vi "generate-folder-name.vi"(7 "vi path base":path, 8 "error in":errorcluster, 9 "report file destination base":path, 11 "vi path":path) -> (0 "error out":errorcluster, 1 "html destination":path, 3 "vi path out":path)   [LabVIEW 2014]
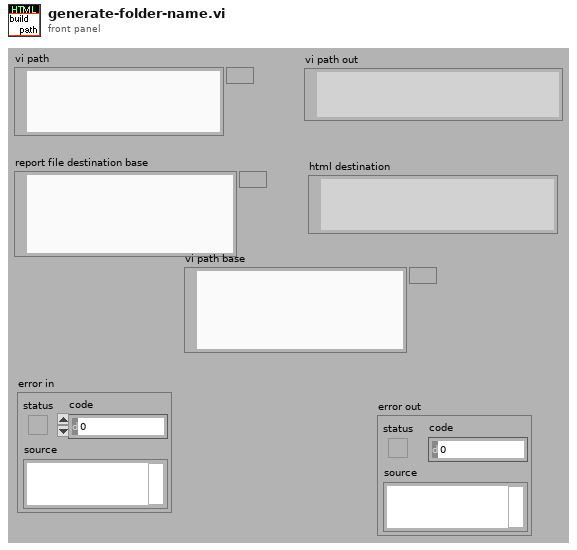
[diagram p1: front panel]
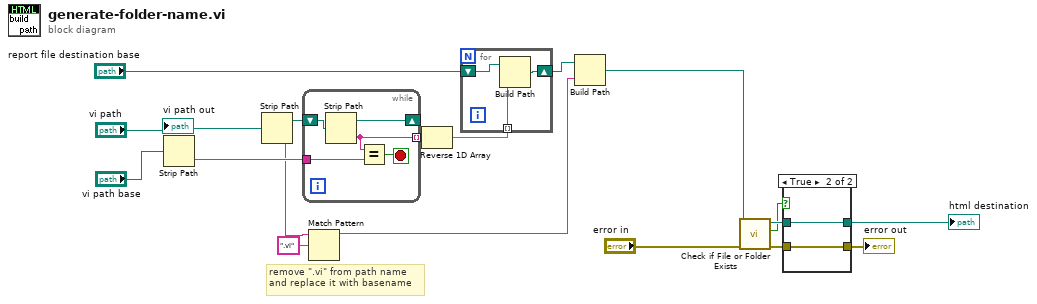
[diagram p0: block diagram]
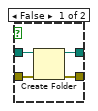
[diagram p2: hidden frame]
diagram:
  # "remove \".vi\" from path name\nand replace it with basename"
  n1 = Strip Path(path="vi path base") -> (name=w12:string)  [unwired: 1 out]
  n2 = Strip Path(path="vi path") -> (stripped path=w9:path, name=w5:string)
  n3 = while {
    shift-right: [w22] -> _
    shift-left: w9 -> [w23]
    tunnel: w12 -> [w21]
    tunnel: [w19] -> w3 mode=indexing
    stop <- w20 stop-if-true
    n4 = Strip Path(path=w23) -> (stripped path=w22:path, name=w19:string)
    n5 = Equal?(x=w19, y=w21) -> (x = y?=w20:bool)
  }
  n6 = Match Pattern(string=w5, regular expression=".vi") -> (before substring=w7:string)  [unwired: 4 out]
  n7 = Reverse 1D Array(array=w3) -> (reversed array=w1:string[])
  n8 = for {
    shift-right: [w25] -> w2
    shift-left: "report file destination base" -> [w26]
    tunnel: w1 -> [w24] mode=indexing
    n9 = Build Path(base path=w26, name or relative path=w24) -> (appended path=w25:path)
  }
  n10 = Build Path(base path=w2, name or relative path=w7) -> (appended path=w8:path)
  n11 = call <vilib>:"Check if File or Folder Exists.vi"("error in (no error)"="error in", "path"=w8) -> ("error out"=w17:errorcluster, "file or folder exists?"=w15:bool, "dup path"=w16:path)  [unwired: 7 out]
  n12 = case shown="True" w15 {
    tunnel: w16 -> [w30 w32]
    tunnel: [w29 w32] -> w14
    tunnel: w17 -> [w28 w31]
    tunnel: [w27 w31] -> w18
    frame False {
      n13 = Create Folder(path (use dialog)=w30, error in=w28) -> (created path=w29:path, error out=w27:errorcluster)  [unwired: 2 out]
    }
    frame True {
    }
  }
  "error out" <- w18
  "html destination" <- w14
  "vi path out" <- "vi path"
